vi "gerador de matriz.vi"(6 "sigma":sgl, 8 "Temperatures":cluster{"Ts":sgl, "Tp":sgl, "Tb":sgl}, 9 "target size":cluster{"sx":i32, "sy":i32}, 10 "target position":cluster{"x":i32, "y":i32}, 11 "Window":cluster{"Rw":i32, "Rh":i32}) -> (1 "error out":errorcluster, 3 "initialized array":sgl[][](array[numeric]))   [LabVIEW 2016]
uses:
  <vilib>/gmath/statdist.llb/Normal Random.vi
  <vilib>/gmath/NI_Gmath.lvlib
panel:
  # "coordenadas do sinalizador (começam do 0),\nrepresentam canto superior esquerdo"
  # "White Gaussian Noise (mu=0)"
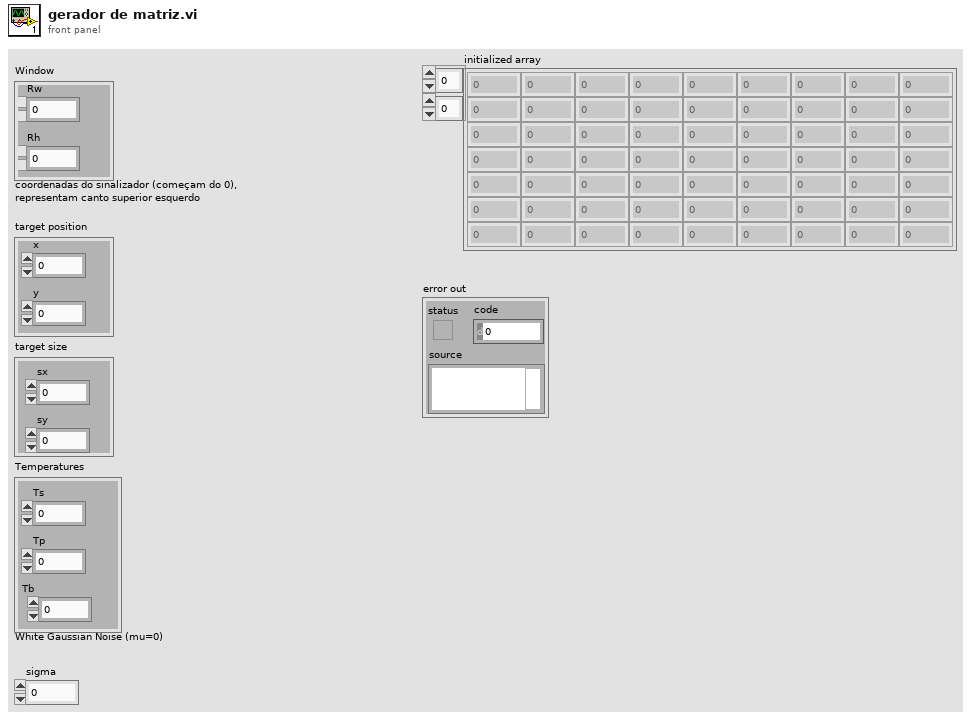
[diagram p1: front panel]
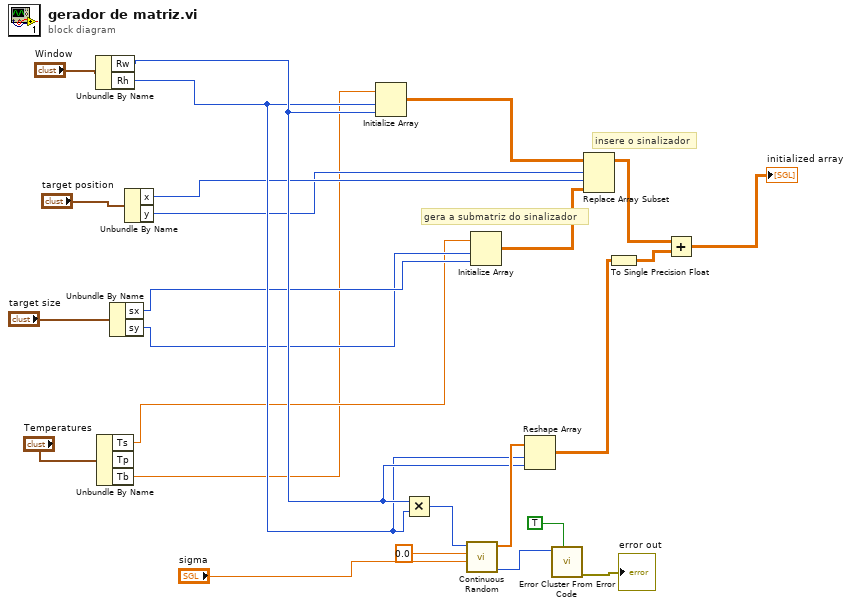
[diagram p0: block diagram]
diagram:
  # "gera a submatriz do sinalizador"
  # "insere o sinalizador"
  n1 = Unbundle By Name("Window") -> ("Rw"=w11:i32, "Rh"=w10:i32)
  n2 = Unbundle By Name("Temperatures") -> ("Ts"=w2:sgl, "Tb"=w1:sgl)  [unwired: 1 out]
  n3 = Unbundle By Name("target size") -> ("sx"=w5:i32, "sy"=w4:i32)
  n4 = Unbundle By Name("target position") -> ("x"=w8:i32, "y"=w7:i32)
  n5 = Initialize Array(w1, w10, w11) -> (w25:sgl[][])
  n6 = Multiply(x=w11, y=w10) -> (x*y=w18:i32)
  n7 = call-poly <vilib>:"Continuous Random.vi"("std"="sigma", "mean"=0.0, "samples"=w18) -> ("error"=w21:i32, "normal random data"=w17:dbl[])  [unwired: 7 in]
  n8 = Initialize Array(w2, w4, w5) -> (w24:sgl[][])
  n9 = Reshape Array(w17, w10, w11) -> (w15:dbl[][])
  n10 = call <vilib>:"Error Cluster From Error Code.vi"("show call chain? (False)"=TRUE, "error code (0)"=w21) -> ("error out"=→"error out":errorcluster)  [unwired: 7 in]
  n11 = Replace Array Subset(array=w25, new element=w24, index (row)=w7, index (col)=w8) -> (w16:sgl[][])
  n12 = To Single Precision Float(number=w15) -> (single precision float=w13:sgl[][])
  n13 = Add(x=w16, y=w13) -> (x+y=→"initialized array":sgl[][])
